vi "Initiate.vi"(8 "error in (no error)":errorcluster, 11 "VISA resource name":refnum<visa-resource-name>) -> (0 "error out":errorcluster, 3 "VISA resource name out":refnum<visa-resource-name>)   [LabVIEW 2024, in "EFmeter.lvlib"]
doc: "This low-level VI initiates a measurement. After you call this VI, the instrument leaves the idle state and waits for a trigger.\n\n<B>Note:</B> Use this VI only with other low-level VIs. The high-level VIs automatically incorporate this functionality. This VI does not check the instrument status. If you want to check the instrument status, call the <B>Error Query</B> VI at the conclusion of the sequence."
uses:
  <instrlib>/EFmeter/EFmeter.lvlib
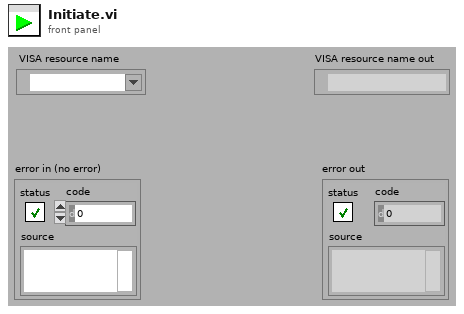
[diagram p1: front panel]
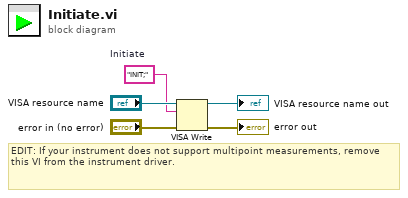
[diagram p0: block diagram]
diagram:
  w3 = "INIT;"  # Initiate
  # "EDIT: If your instrument does not support multipoint measurements, remove this VI from the instrument driver."
  n1 = VISA Write(VISA resource name="VISA resource name", write buffer=w3, error in (no error)="error in (no error)") -> (VISA resource name out=→"VISA resource name out":refnum<visa-resource-name>, error out=→"error out":errorcluster)  [unwired: 1 out]
